vi "Verify.vi"(8 "error in":errorcluster, 10 "Test Data":string) -> (0 "error out":errorcluster)   [LabVIEW 2020, in "Caraya.Extension.lvlib"]
uses:
  Caraya.Extension.lvlib
  <vilib>/addons/_JKI Toolkits/Caraya/classes/Assert/Assert True.vi
  Approval Tests/Approval Tests.lvlib
  <vilib>/addons/_JKI Toolkits/Caraya/classes/Assert/Assert.lvclass
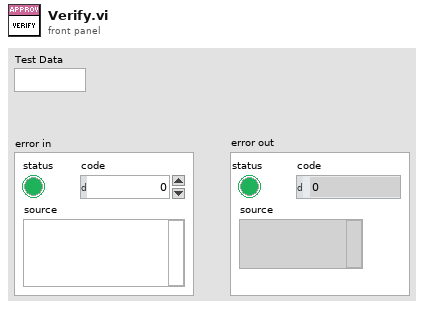
[diagram p1: front panel]
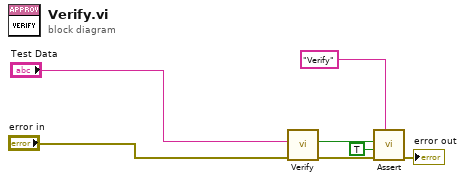
[diagram p0: block diagram]
diagram:
  n1 = call "Verify.vi"("error in"="error in", "Test Data"="Test Data") -> ("error out"=w6:errorcluster, "Passed?"=w1:bool)  [unwired: 7 in, 1 out]
  n2 = call-poly <vilib>:"Assert.vi"("Label"="Verify", "error in (no error)"=w6, "Register with caller test (F)"=TRUE, "True?"=w1) -> ("error out"=→"error out":errorcluster)  [unwired: 6 in, 1 out]
